vi "Open Session.vi"(8 "error in (no error)":errorcluster, 11 "Serial Session in":refnum<class "Serial Session.lvclass">) -> (0 "error out":errorcluster, 3 "Serial Session out":refnum<class "Serial Session.lvclass">)   [LabVIEW 2016, in "Serial Session.lvclass"]
doc: "This method is simply a wrapper for the VISA Open method. Wrapping this here allows to break out the configuration process and extend the class for use with other types of interfaces besides RS232 (i.e. GPIB). In the latter case, we may not desire to utilize all of the configuration options available with serial sessions and we simply want to open a port. This allows the user to instatiate without having to perform a full on configuration of the port."
uses:
  Serial Session.lvclass
  Serial Session.lvclass/Serial Session.ctl
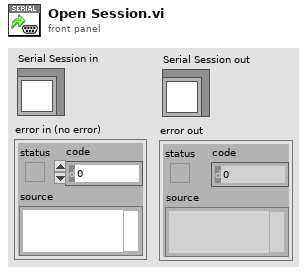
[diagram p1: front panel]
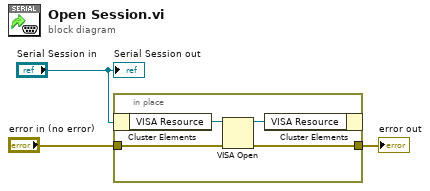
[diagram p0: block diagram]
diagram:
  n1 = in-place {
    in-place-border: "error in (no error)" -> [w7]
    in-place-border: [w6] -> w2
    n2 = in-place-cluster #1("Serial Session in") -> ("VISA Resource"=w5:refnum<visa-resource-name>)
    n3 = VISA Open(error in (no error)=w7, VISA resource name=w5) -> (VISA resource name=w4:refnum<visa-resource-name>, error out=w6:errorcluster)  [unwired: 3 in]
    n4 = in-place-cluster #1("VISA Resource"=w4) -> ()  [unwired: 1 out]
  }
  "error out" <- w2
  "Serial Session out" <- "Serial Session in"
